vi "Initialize Endpoint Configuration Page.vi"(8 "error in (no error)":errorcluster, 10 "Endpoint Configuration Page Controls":T1, 11 "Node Ptr":T2 format="%.0x") -> (0 "error out":errorcluster, 3 "Endpoint Configuration Section Ref out":T2 format="%.0x")   [LabVIEW 2017, in "NI-SWITCH System Explorer.lvlib"]
uses:
  NI-SWITCH System Explorer.lvlib
  <vilib>/NI Veristand/Custom Device API/Custom Device Item Ref.ctl
  Endpoint Configuration Page Controls.ctl
  Shared/UI Common/Sort Button.ctl
  Scripting/NI-SWITCH Scripting.lvlib
  <vilib>/NI VeriStand/Custom Device API/Custom Device API.lvlib
  Shared/UI Common/UI Common.lvlib
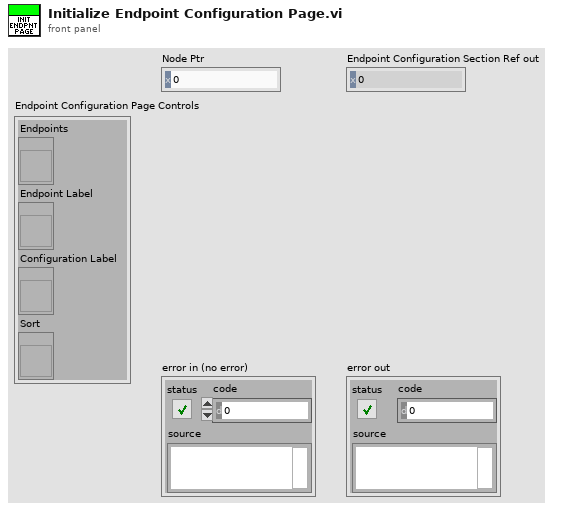
[diagram p1: front panel]
types:
  T1 = typedef "NI-SWITCH System Explorer.lvlib/Endpoint Configuration Page Controls.ctl" = cluster{"Endpoints":refnum<vi>, "Endpoint Label":refnum<vi>, "Configuration Label":refnum<vi>, "Sort":refnum<vi>}
  T2 = typedef "Custom Device API.lvlib/Custom Device Item Ref.ctl" = u64
  T3 = enum8{"Enabled", "Disabled", "Disabled and Grayed Out"}
  T4 = typedef "NI-SWITCH Shared.lvlib/Endpoint Configuration Cluster.ctl" = cluster{"Endpoint":string, "Configuration":T5}
  T5 = typedef "NI-SWITCH Shared.lvlib/Endpoint Configuration Enum.ctl" = enum16{"Load", "Source", "Configuration"}
  T6 = typedef "NI-SWITCH System Explorer.lvlib/Channel.ctl" = cluster{"Endpoint":string, "Configuration":T7}
  T7 = typedef "NI-SWITCH System Explorer.lvlib/Channel Type.ctl" = enum16{"Load (Default)", "Source", "Configuration"}
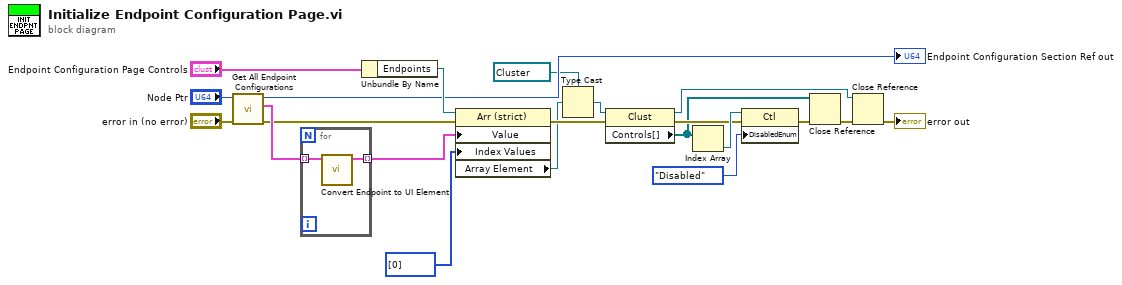
[diagram p0: block diagram]
diagram:
  n1 = call "Get All Endpoint Configurations.vi"("error in"="error in (no error)", "endpoint configuration in"="Node Ptr") -> ("error out"=w14:errorcluster, "endpoint configurations"=w21:T4[], "endpoint configuration out"=→"Endpoint Configuration Section Ref out":T2)  [unwired: 7 in]
  n2 = for {
    tunnel: w21 -> [w22] mode=indexing
    tunnel: [w23] -> w16 mode=indexing
    n3 = call "Convert Endpoint to UI Element.vi"("Connection"=w22) -> ("Channel"=w23:T6)  [unwired: 10 in]
  }
  n4 = Unbundle By Name("Endpoint Configuration Page Controls") -> ("Endpoints"=w17:refnum<vi>)
  n5 = property class="Arr (strict)"(reference=w17, error in=w14, "Value"=w16, "Index Values"=u32[] [0]) -> (error out=w9:errorcluster, "Array Element"=w7:refnum<vi>)  [unwired: 1 out]
  n6 = Type Cast(type=refnum<vi> refnum ("Array Element"), x=w7) -> (*(type *) &x=w6:refnum<vi>)
  n7 = property class="Clust"(reference=w6, error in=w9) -> (reference out=w1:refnum<vi>, error out=w10:errorcluster, "Controls[]"=w4:refnum<vi>[])
  n8 = Index Array(array=w4) -> (element=w12:refnum<vi>)  [unwired: 1 in]
  n9 = property class="Ctl"(reference=w12, error in=w10, "DisabledEnum"=T3."Disabled" ("Disabled")) -> (error out=w5:errorcluster)  [unwired: 1 out]
  n10 = Close Reference(reference=w4, error in (no error)=w5) -> (error out=w3:errorcluster)
  n11 = Close Reference(reference=w1, error in (no error)=w3) -> (error out=→"error out":errorcluster)
